vi "RxBfrPkt - Add Channels.vi"(7 "Ext Buffer?":bool, 8 "error in (no error)":errorcluster, 11 "Node Ptr":T1 format="%.0x") -> (0 "error out":errorcluster, 3 "Node Ptr out":T1 format="%.0x")   [LabVIEW 2019, in "UDP-Custom-Device System Explorer.lvlib"]
uses:
  UDP-Custom-Device System Explorer.lvlib
  <vilib>/NI VeriStand/Custom Device API/Custom Device Item Ref.ctl
  <vilib>/NI VeriStand/Custom Device API/Custom Device Channel.ctl
  <vilib>/NI VeriStand/Custom Device API/Custom Device Channel Type.ctl
  <vilib>/NI VeriStand/Custom Device API/Custom Device API.lvlib
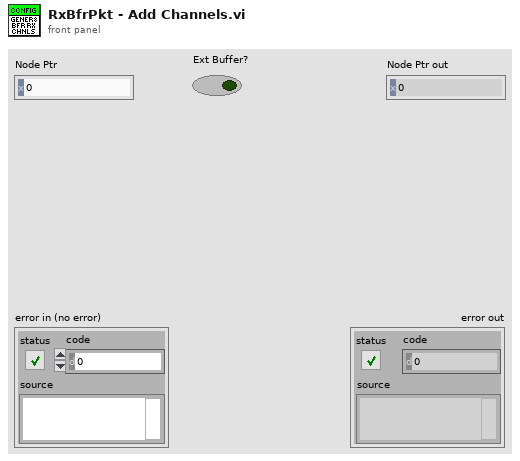
[diagram p1: front panel]
types:
  T1 = typedef "Custom Device API.lvlib/Custom Device Item Ref.ctl" = u64
  T2 = typedef "Custom Device API.lvlib/Custom Device Channel Type.ctl" = enum16{"Input", "Output"}
  T3 = typedef "Custom Device API.lvlib/Custom Device Channel.ctl" = cluster{"Type":T2, "Units":string, "Default Value":dbl, "Faultable":bool, "Scalable":bool}
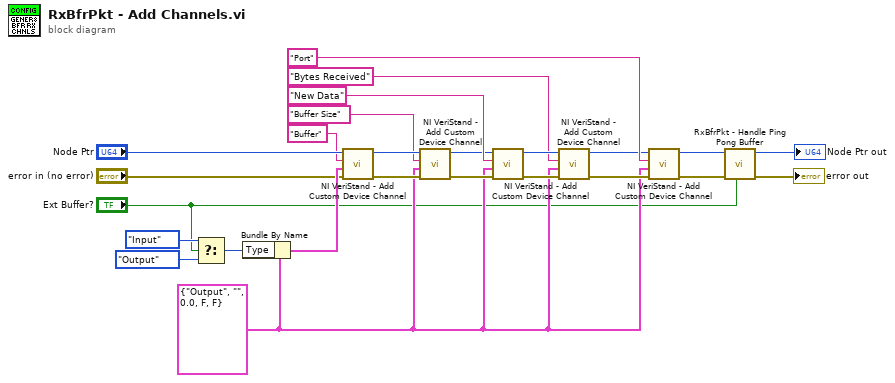
[diagram p0: block diagram]
diagram:
  w6 = T3 {"Type"=enum."Output", "Units"="", "Default Value"=0.0, "Faultable"=FALSE, "Scalable"=FALSE} ("Channel")
  n1 = Select(t=Custom_Device_Channel_Type."Input" ("Type"), s="Ext Buffer?", f=Custom_Device_Channel_Type."Output" ("Type")) -> (s? t:f=w15:T2)
  n2 = Bundle By Name(cluster=w6, "Type"=w15) -> (w14:T3)
  n3 = call <vilib>:"NI VeriStand - Add Custom Device Channel.vi"("error in (no error)"="error in (no error)", "Channel"=w14, "Channel Name"="Buffer", "Parent Ref in"="Node Ptr") -> ("error out"=w9:errorcluster, "Parent Ref out"=w11:T1)  [unwired: 4 in, 2 out]
  n4 = call <vilib>:"NI VeriStand - Add Custom Device Channel.vi"("error in (no error)"=w9, "Channel"=w6, "Channel Name"="Buffer Size", "Parent Ref in"=w11) -> ("error out"=w8:errorcluster, "Parent Ref out"=w10:T1)  [unwired: 4 in, 2 out]
  n5 = call <vilib>:"NI VeriStand - Add Custom Device Channel.vi"("error in (no error)"=w8, "Channel"=w6, "Channel Name"="New Data", "Parent Ref in"=w10) -> ("error out"=w23:errorcluster, "Parent Ref out"=w24:T1)  [unwired: 4 in, 2 out]
  n6 = call <vilib>:"NI VeriStand - Add Custom Device Channel.vi"("error in (no error)"=w23, "Channel"=w6, "Channel Name"="Bytes Received", "Parent Ref in"=w24) -> ("error out"=w20:errorcluster, "Parent Ref out"=w19:T1)  [unwired: 4 in, 2 out]
  n7 = call <vilib>:"NI VeriStand - Add Custom Device Channel.vi"("error in (no error)"=w20, "Channel"=w6, "Channel Name"="Port", "Parent Ref in"=w19) -> ("error out"=w5:errorcluster, "Parent Ref out"=w3:T1)  [unwired: 4 in, 2 out]
  n8 = call "RxBfrPkt - Handle Ping Pong Buffer.vi"("Ext Buffer?"="Ext Buffer?", "error in (no error)"=w5, "Node Ptr"=w3) -> ("error out"=→"error out":errorcluster, "Node Ptr out"=→"Node Ptr out":T1)  [unwired: 7 in]
